vi "DMM Configuration.vi"(8 "error in (no error)":errorcluster, 11 "Node Ptr":T1 format="%.0x") -> (0 "error out":errorcluster)   [LabVIEW 2015, in "DMM-SWITCH-ScanList System Explorer.lvlib"]
uses:
  DMM-SWITCH-ScanList System Explorer.lvlib
  <vilib>/NI Veristand/Custom Device API/Custom Device Item Ref.ctl
  Shared/Constants.vi
  <vilib>/NI Veristand/Custom Device API/Get Item Property (U16).vi
  <vilib>/NI Veristand/Custom Device API/Get Item Property (Double).vi
  <vilib>/NI Veristand/Custom Device API/Get Item Property (String).vi
  <vilib>/NI Veristand/Custom Device API/Set Item Property (String).vi
  <vilib>/NI Veristand/Custom Device API/Set Item Property (Double).vi
  <vilib>/NI Veristand/Custom Device API/Set Item Property (U16).vi
  <vilib>/NI Veristand/Custom Device API/Custom Device API.lvlib
  Shared/DMM-SWITCH-ScanList Shared.lvlib
panel:
  in  "Range":u16(ring)
  in  "Resolution in Digits":u16(ring)
  in  "Measurements":u16(ring)
  in  "DMM Resource Name":string
  in  "Header":cluster{"Section Name":string}={"Section Name"="Custom Device Item Settings"}
  in  "Description":string
  in  "Name":string
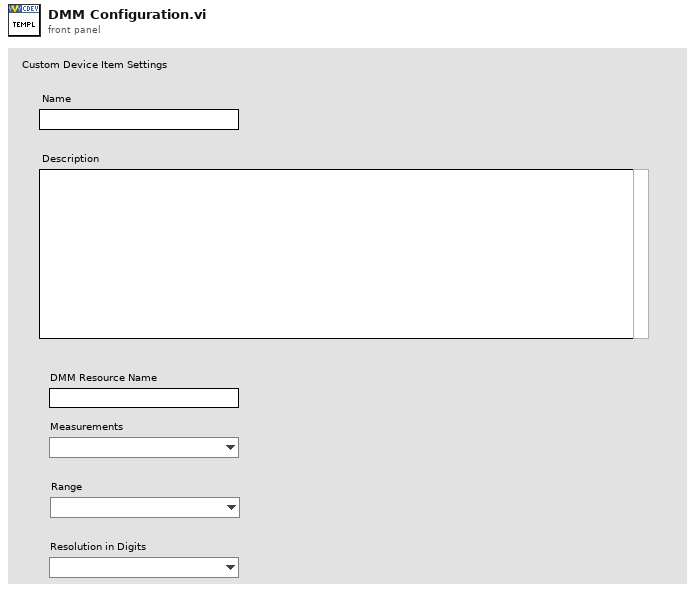
[diagram p1: front panel]
types:
  T1 = typedef "Custom Device API.lvlib/Custom Device Item Ref.ctl" = u64
  T2 = typedef "Custom Device API.lvlib/Custom Device Item Info.ctl" = cluster{"Name":string, "Is Channel":bool, "GUID":string, "Is Waveform":bool}
  T3 = typedef "Custom Device API.lvlib/Custom Device Commands.ctl" = enum16{"Default", "Item renamed", "Shutdown", "Dynamic button pressed"}
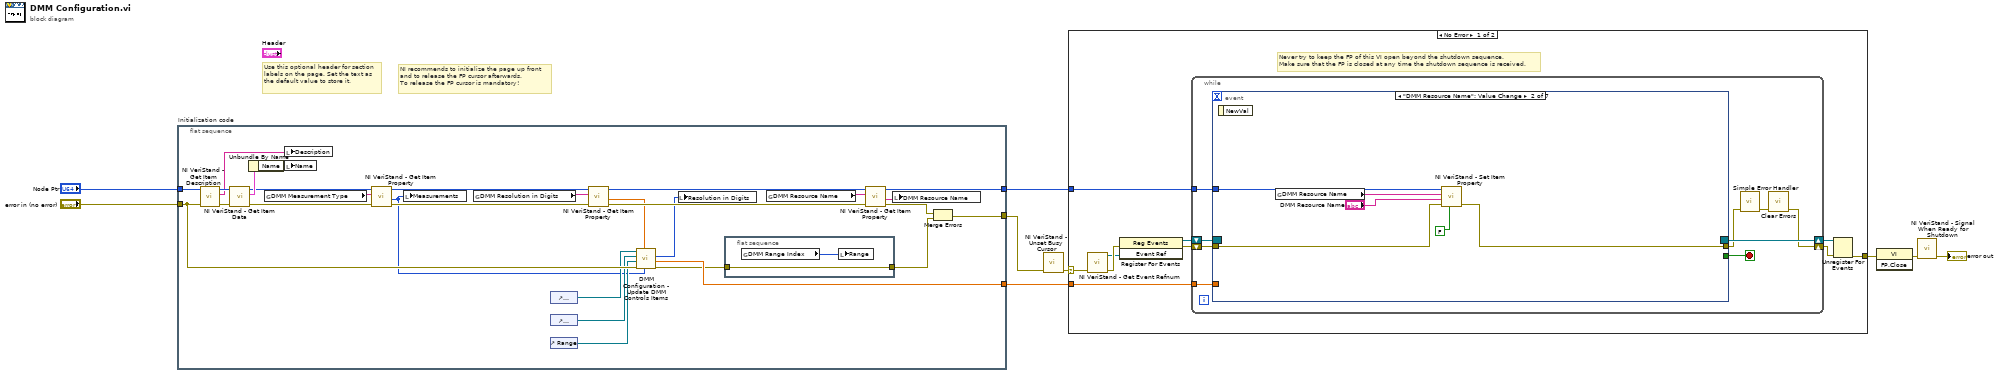
[diagram p0: block diagram]
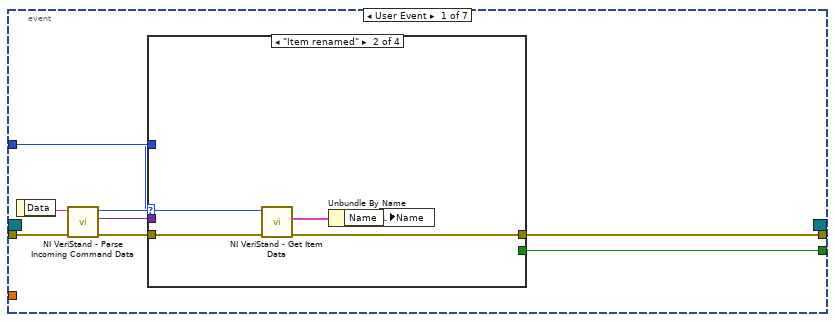
[diagram p2: hidden frame]
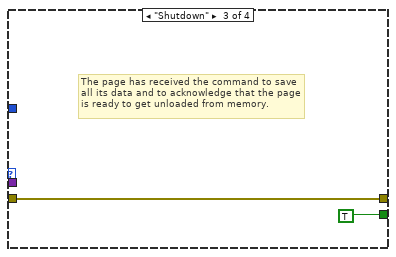
[diagram p4: hidden frame]
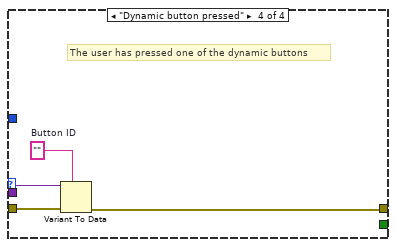
[diagram p5: hidden frame]
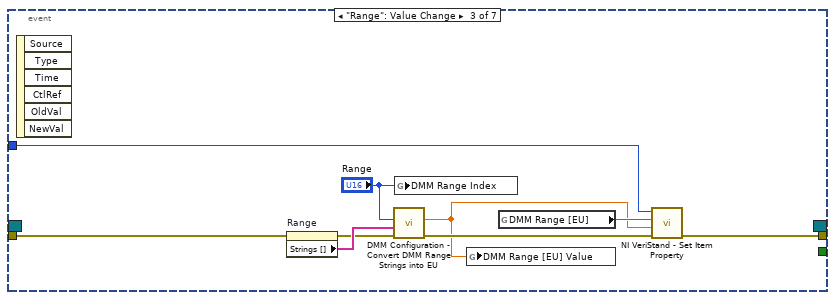
[diagram p6: hidden frame]
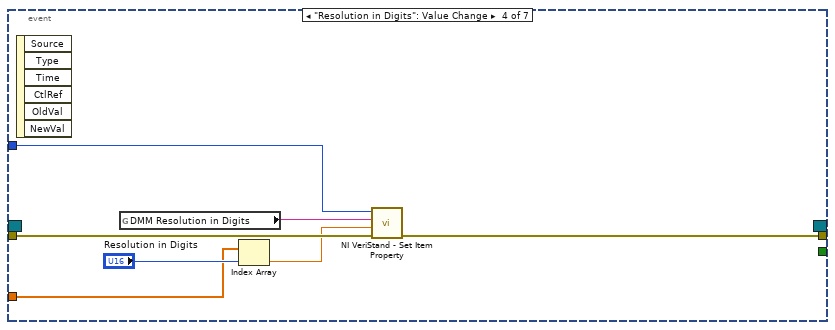
[diagram p7: hidden frame]
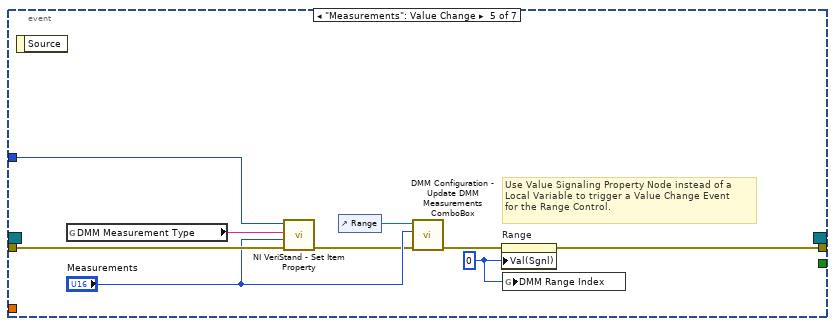
[diagram p8: hidden frame]
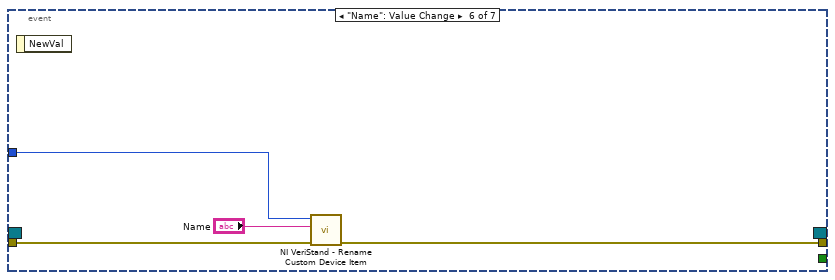
[diagram p9: hidden frame]
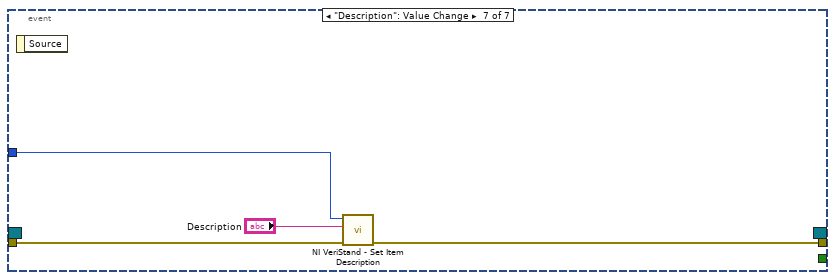
[diagram p10: hidden frame]
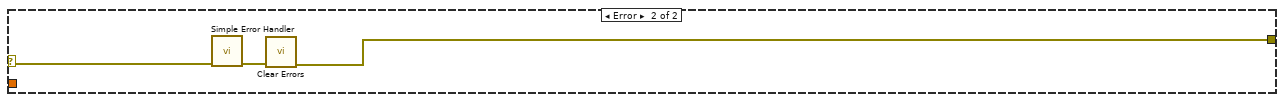
[diagram p11: hidden frame]
diagram:
  # "Use this optional header for section labels on the page. Set the text as the default value to store it."
  # "NI recommends to initialize the page up front\nand to release the FP cursor afterwards.\nTo release the FP cursor is mandatory!"
  n1 = flat-sequence "Initialization code" {
    tunnel: "error in (no error)" -> [w18]
    tunnel: "Node Ptr" -> [w37]
    tunnel: [w23] -> w5
    tunnel: [w27] -> w2
    tunnel: [w11] -> w1
    frame #0 {
      n2 = call <vilib>:"NI VeriStand - Get Item Description.vi"("error in (no error)"=w18, "Item Ref in"=w37) -> ("error out"=w35:errorcluster, "Description"=w36:string, "Item Ref out"=w38:T1)  [unwired: 7 out]
      n3 = call <vilib>:"NI VeriStand - Get Item Data.vi"("error in (no error)"=w35, "Item Ref in"=w38) -> ("error out"=w32:errorcluster, "Item Info"=w34:T2, "Item Ref out"=w31:T1)  [unwired: 7 out]
      n4 = Unbundle By Name(w34) -> ("Name"=w33:string)
      n5 = global read "Constants.vi" "DMM Measurement Type"() -> (w22:string)
      n6 = local write "Description"(w36) -> ()
      n7 = local write "Name"(w33) -> ()
      n8 = call-poly <vilib>:"NI VeriStand - Get Item Property.vi"("error in (no error)"=w32, "Property Name"=w22, "Item Ref in"=w31) -> ("error out"=w29:errorcluster, "Value"=w13:u16, "Item Ref out"=w30:T1)  [unwired: 5 in, 1 out]
      n9 = local write "Measurements"(w13) -> ()
      n10 = global read "Constants.vi" "DMM Resolution in Digits"() -> (w26:string)
      n11 = control-ref of="Measurements"() -> (w17:refnum<vi>)
      n12 = control-ref of="Resolution in Digits"() -> (w16:refnum<vi>)
      n13 = control-ref of="Range"() -> (w15:refnum<vi>)
      n14 = call-poly <vilib>:"NI VeriStand - Get Item Property.vi"("error in (no error)"=w29, "Property Name"=w26, "Item Ref in"=w30) -> ("error out"=w21:errorcluster, "Value"=w14:dbl, "Item Ref out"=w20:T1)  [unwired: 5 in, 1 out]
      n15 = call "DMM Configuration - Update DMM Controls Items.vi"("Measurement In"=w13, "Resolution in Digits Saved Value"=w14, "error in (no error)"=w18, "Range Ref"=w15, "Resoultion in Digits Ref"=w16, "Measurements Ref"=w17) -> ("error out"=w10:errorcluster, "Resolution in Digits Array Out"=w11:dbl[], "Resolution in Digits Index"=w12:i32)  [unwired: 3 in]
      n16 = local write "Resolution in Digits"(w12) -> ()
      n17 = flat-sequence {
        tunnel: w10 -> [w39]
        tunnel: [w39] -> w19
        frame #0 {
          n18 = global read "Constants.vi" "DMM Range Index"() -> (w40:u16)
          n19 = local write "Range"(w40) -> ()
        }
      }
      n20 = global read "Constants.vi" "DMM Resource Name"() -> (w25:string)
      n21 = call-poly <vilib>:"NI VeriStand - Get Item Property.vi"("error in (no error)"=w21, "Property Name"=w25, "Item Ref in"=w20) -> ("error out"=w24:errorcluster, "Value"=w28:string, "Item Ref out"=w27:T1)  [unwired: 5 in, 1 out]
      n22 = local write "DMM Resource Name"(w28) -> ()
      n23 = Merge Errors(w24, w19) -> (w23:errorcluster)
    }
  }
  n24 = call <vilib>:"NI VeriStand - Unset Busy Cursor.vi"("error in (no error)"=w5) -> ("error out"=w4:errorcluster)  [unwired: 10 out]
  n25 = case shown="No Error" w4 {
    selector: w4 -> [w42 w121]
    tunnel: [w47 w119] -> w9
    tunnel: w2 -> [w43 _]
    tunnel: w1 -> [w41 _]
    frame No Error {
      # "Never try to keep the FP of this VI open beyond the shutdown sequence.\nMake sure that the FP is closed at any time the shutdown sequence is received."
      n26 = call <vilib>:"NI VeriStand - Get Event Refnum.vi"("error in (no error)"=w42) -> ("error out"=w50:errorcluster, "Event Ref"=w46:refnum<user-event>)  [unwired: 9 out]
      n27 = register-events(error in=w50, w46) -> (reference out=w44:refnum<event-registration>, error out=w45:errorcluster)  [unwired: 1 in]
      n28 = while {
        tunnel: w43 -> [w55]
        shift-right: [w52] -> w48
        shift-left: w45 -> [w58]
        shift-right: [w59] -> w49
        shift-left: w44 -> [w57]
        tunnel: w41 -> [w51]
        stop <- w56 stop-if-true
        n29 = event shown="[1] \"DMM Resource Name\": Value Change" {
          selector: w57 -> [_ _ _ _ _ _ _]
          dyn-events: [_ _ _ _ _ _ _] -> w59
          timeout: _ -> [_ _ _ _ _ _ _]
          tunnel: w58 -> [w67 w84 w92 w100 w109 w114 w117]
          tunnel: [w63 _ _ _ _ _ _] -> w56
          tunnel: [w62 w83 w94 w99 w106 w113 w116] -> w54
          tunnel: w55 -> [w61 w85 w91 w101 w110 w112 w118]
          tunnel: w51 -> [_ _ _ w95 _ _ _]
          event User Event {
            n30 = event-data() -> ("Data"=w66:string)  [unwired: 1 out]
            n31 = call <vilib>:"NI VeriStand - Parse Incoming Command Data.vi"("error in (no error)"=w67, "Incoming data"=w66) -> ("error out"=w65:errorcluster, "Outgoing data"=w60:variant, "Action"=w64:T3)  [unwired: 7 out]
            n32 = case shown="\"Item renamed\"" w64 {
              tunnel: w65 -> [w68 w73 w74 w79]
              tunnel: [_ _ TRUE _] -> w63
              tunnel: [w68 w70 w74 w76] -> w62
              tunnel: w61 -> [_ w72 _ _]
              tunnel: w60 -> [_ _ _ w78]
              frame "Default", Default {
              }
              frame "Item renamed" {
                n33 = call <vilib>:"NI VeriStand - Get Item Data.vi"("error in (no error)"=w73, "Item Ref in"=w72) -> ("error out"=w70:errorcluster, "Item Info"=w71:T2)  [unwired: 8 out]
                n34 = Unbundle By Name(w71) -> ("Name"=w69:string)
                n35 = local write "Name"(w69) -> ()
              }
              frame "Shutdown" {
                # "The page has received the command to save all its data and to acknowledge that the page is ready to get unloaded from memory."
              }
              frame "Dynamic button pressed" {
                w77 = ""  # Button ID
                # "The user has pressed one of the dynamic buttons"
                n36 = Variant To Data(error in=w79, type=w77, Variant=w78) -> (error out=w76:errorcluster)  [unwired: 1 out]
              }
            }
          }
          event "DMM Resource Name": Value Change {
            n37 = event-data() -> ()  [unwired: 2 out]
            n38 = global read "Constants.vi" "DMM Resource Name"() -> (w80:string)
            n39 = call-poly <vilib>:"NI VeriStand - Set Item Property.vi"("Binary String (T)"=FALSE, "error in (no error)"=w84, "Value"="DMM Resource Name", "Property Name"=w80, "Item Ref in"=w85) -> ("error out"=w83:errorcluster)  [unwired: 4 in, 2 out]
          }
          event "Range": Value Change {
            n40 = event-data() -> ()  [unwired: 7 out]
            n41 = property on="Range" class="Ring (strict)"(error in=w92) -> (error out=w88:errorcluster, "Strings []"=w89:string[])  [unwired: 1 in, 1 out]
            n42 = call "DMM Configuration - Convert DMM Range Strings into EU.vi"("error in (no error)"=w88, "DMM Range ComboBox Strings"=w89, "Dmm Range Index In"="Range") -> ("error out"=w87:errorcluster, "DMM Range [EU]"=w86:dbl)  [unwired: 7 in]
            n43 = global write "Constants.vi" "DMM Range Index"("Range") -> ()
            n44 = global write "Constants.vi" "DMM Range [EU] Value"(w86) -> ()
            n45 = global read "Constants.vi" "DMM Range [EU]"() -> (w93:string)
            n46 = call-poly <vilib>:"NI VeriStand - Set Item Property.vi"("error in (no error)"=w87, "Value"=w86, "Property Name"=w93, "Item Ref in"=w91) -> ("error out"=w94:errorcluster)  [unwired: 5 in, 2 out]
          }
          event "Resolution in Digits": Value Change {
            n47 = event-data() -> ()  [unwired: 7 out]
            n48 = global read "Constants.vi" "DMM Resolution in Digits"() -> (w98:string)
            n49 = Index Array(array=w95, index="Resolution in Digits") -> (element=w97:dbl)
            n50 = call-poly <vilib>:"NI VeriStand - Set Item Property.vi"("error in (no error)"=w100, "Value"=w97, "Property Name"=w98, "Item Ref in"=w101) -> ("error out"=w99:errorcluster)  [unwired: 5 in, 2 out]
          }
          event "Measurements": Value Change {
            w107 = 0
            # "Use Value Signaling Property Node instead of a \nLocal Variable to trigger a Value Change Event \nfor the Range Control."
            n51 = event-data() -> ()  [unwired: 2 out]
            n52 = global read "Constants.vi" "DMM Measurement Type"() -> (w108:string)
            n53 = call-poly <vilib>:"NI VeriStand - Set Item Property.vi"("error in (no error)"=w109, "Value"="Measurements", "Property Name"=w108, "Item Ref in"=w110) -> ("error out"=w103:errorcluster)  [unwired: 5 in, 2 out]
            n54 = control-ref of="Range"() -> (w105:refnum<vi>)
            n55 = call "DMM Configuration - Update DMM Measurements ComboBox.vi"("error in (no error)"=w103, "Measurement"="Measurements", "Ring in"=w105) -> ("error out"=w102:errorcluster)  [unwired: 8 in]
            n56 = property on="Range" class="Ring (strict)"(error in=w102, "Val(Sgnl)"=w107) -> (error out=w106:errorcluster)  [unwired: 1 in, 1 out]
            n57 = global write "Constants.vi" "DMM Range Index"(w107) -> ()
          }
          event "Name": Value Change {
            n58 = event-data() -> ()  [unwired: 2 out]
            n59 = call <vilib>:"NI VeriStand - Rename Custom Device Item.vi"("error in (no error)"=w114, "New Name"="Name", "Item Ref in"=w112) -> ("error out"=w113:errorcluster)  [unwired: 1 in, 7 out]
          }
          event "Description": Value Change {
            n60 = event-data() -> ()  [unwired: 2 out]
            n61 = call <vilib>:"NI VeriStand - Set Item Description.vi"("error in (no error)"=w117, "Description"="Description", "Item Ref in"=w118) -> ("error out"=w116:errorcluster)  [unwired: 8 out]
          }
        }
        n62 = call <vilib>:"Simple Error Handler.vi"("error in (no error)"=w54) -> ("error out"=w53:errorcluster)  [unwired: 1 in, 7 out]
        n63 = call <vilib>:"Clear Errors.vi"("error in (no error)"=w53) -> ("error out"=w52:errorcluster)  [unwired: 1 in, 5 out]
      }
      n64 = Unregister For Events(event registration refnum=w49, error in=w48) -> (error out=w47:errorcluster)
    }
    frame Error {
      n65 = call <vilib>:"Simple Error Handler.vi"("error in (no error)"=w121) -> ("error out"=w120:errorcluster)  [unwired: 1 in, 7 out]
      n66 = call <vilib>:"Clear Errors.vi"("error in (no error)"=w120) -> ("error out"=w119:errorcluster)  [unwired: 1 in, 5 out]
    }
  }
  n67 = invoke class="VI" method="FP.Close"(error in=w9) -> (error out=w8:errorcluster)  [unwired: 2 in, 2 out]
  n68 = call <vilib>:"NI VeriStand - Signal When Ready for Shutdown.vi"("error in (no error)"=w8) -> ("error out"=→"error out":errorcluster)  [unwired: 10 out]
